vi "LocallyLinearEmbedding.vi"(8 "error in":errorcluster) -> (0 "error out":errorcluster, 3 "out":refnum<class "LocallyLinearEmbedding.lvclass">)   [LabVIEW 2020]
doc: "Locally Linear Embedding\n\n Read more in the :ref:`User Guide <locally_linear_embedding>`.\n\n Parameters\n ----------\n n_neighbors : int, default=5\n number of neighbors to consider for each point.\n\n n_components : int, default=2\n number of coordinates for the manifold\n\n reg : float, default=1e-3\n regularization constant, multiplies the trace of the local covariance\n matrix of the distances.\n\n eigen_solver : {'auto', 'arpack', 'dense'}, default='auto'\n auto : algorithm will attempt to choose the best method for input data\n\n arpack : use arnoldi iteration in shift-invert mode.\n For this method, M may be a dense matrix, sparse matrix,\n or general linear operator.\n Warning: ARPACK can be unstable for some problems. It is\n best to try several random seeds in order to check results.\n\n dense : use standard dense matrix operations for the eigenvalue\n decomposition. For this method, M must be an array\n or matrix type. This method should be avoided for\n large problems.\n\n tol : float, default=1e-6\n Tolerance for 'arpack' method\n Not used if eigen_solver=='dense'.\n\n max_iter : int, default=100\n maximum number of iterations for the arpack solver.\n Not used if eigen_solver=='dense'.\n\n method : {'standard', 'hessian', 'modified', 'ltsa'}, default='standard'\n - `standard`: use the standard locally linear embedding algorithm. see\n reference [1]_\n - `hessian`: use the Hessian eigenmap method. This method requires\n ``n_neighbors > n_components * (1 + (n_components + 1) / 2``. see\n reference [2]_\n - `modified`: use the modified locally linear embedding algorithm.\n see reference [3]_\n - `ltsa`: use local tangent space alignment algorithm. see\n reference [4]_\n\n hessian_tol : float, default=1e-4\n Tolerance for Hessian eigenmapping method.\n Only used if ``method == 'hessian'``\n\n modified_tol : float, default=1e-12\n Tolerance for modified LLE method.\n Only used if ``method == 'modified'``\n\n neighbors_algorithm : {'auto', 'brute', 'kd_tree', 'ball_tree'}, default='auto'\n algorithm to use for nearest neighbors search,\n passed to neighbors.NearestNeighbors instance\n\n random_state : int, RandomState instance, default=None\n Determines the random number generator when\n ``eigen_solver`` == 'arpack'. Pass an int for reproducible results\n across multiple function calls. See :term: `Glossary <random_state>`.\n\n n_jobs : int or None, default=None\n The number of parallel jobs to run.\n ``None`` means 1 unless in a :obj:`joblib.parallel_backend` context.\n ``-1`` means using all processors. See :term:`Glossary <n_jobs>`\n for more details.\n\n Attributes\n ----------\n embedding_ : array-like, shape [n_samples, n_components]\n Stores the embedding vectors\n\n reconstruction_error_ : float\n Reconstruction error associated with `embedding_`\n\n nbrs_ : NearestNeighbors object\n Stores nearest neighbors instance, including BallTree or KDtree\n if applicable.\n\n \nAvailable methods:\nFit\nFit Transform\nGet Attributes\nGet Params\nSet Params"
uses:
  LocallyLinearEmbedding.lvclass
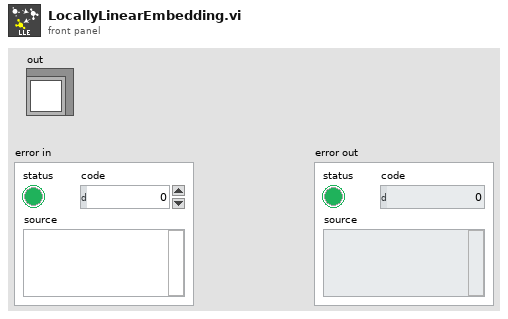
[diagram p1: front panel]
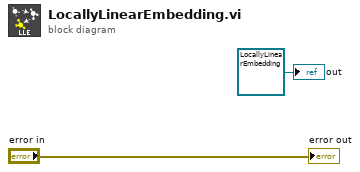
[diagram p0: block diagram]
diagram:
  "out" <- refnum<class "LocallyLinearEmbedding.lvclass"> refnum ("model")
  "error out" <- "error in"
